vi "Read Message.vi"(8 "error in (no error)":errorcluster, 11 "_Popup in":refnum<class "Popup.lvclass">) -> (0 "error out":errorcluster, 2 "Message":string, 3 "_Popup out":refnum<class "Popup.lvclass">)   [LabVIEW 2021, in "Pop-Up.lvlib" / "Popup.lvclass"]
doc: "This Data Member Access VI will read the Label from the object.\n\nOutputs: +\n-Label [string] - label string to write to the pop up display\n\n<b>Code Developed By:</b> +\nDaniel Coons +\nhttps://github.com/danielcoons/tsc-pop-up"
uses:
  Popup.lvclass
  Popup.lvclass/Popup.ctl
panel:
  # "This VI gets the label value (string) from the Popup Object"
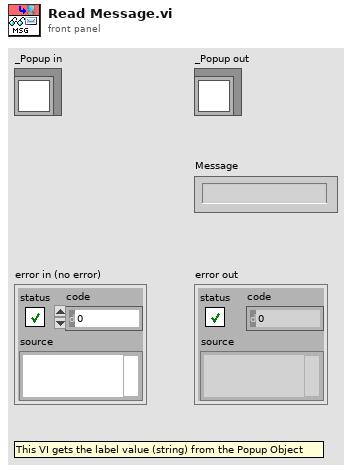
[diagram p1: front panel]
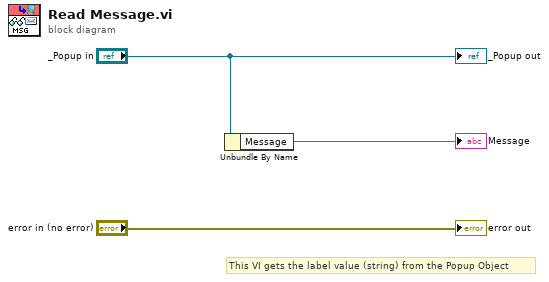
[diagram p0: block diagram]
diagram:
  # "This VI gets the label value (string) from the Popup Object"
  n1 = Unbundle By Name("_Popup in") -> ("Message"=→"Message":string)
  "error out" <- "error in (no error)"
  "_Popup out" <- "_Popup in"
